vi "pressure_calibration.vi"(10 "calibration":T1(ring), 11 "cmd pressure (mBar)":dbl format="%#_13g") -> (3 "pressure out (mbar)":dbl format="%#_13g")   [LabVIEW 2019]
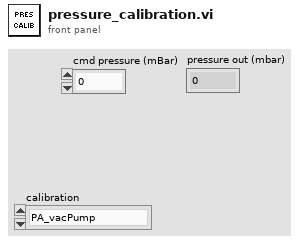
[diagram p1: front panel]
types:
  T1 = enum16{"PA_vacPump", "PA_venturi", "Neuromatics", "ilyaRig", "mightenRig"}
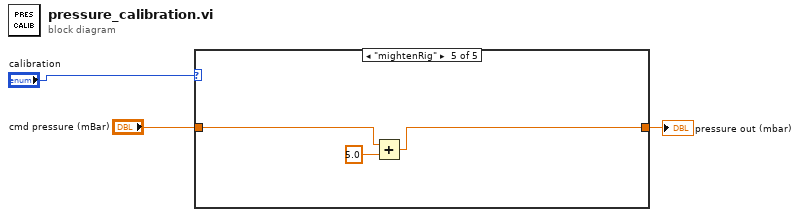
[diagram p0: block diagram]
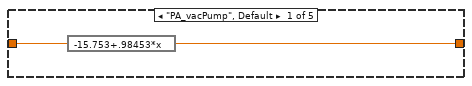
[diagram p2: hidden frame]
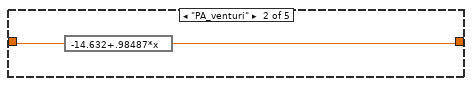
[diagram p3: hidden frame]
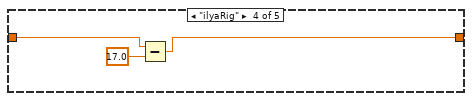
[diagram p5: hidden frame]
diagram:
  n1 = case shown="\"mightenRig\"" "calibration" {
    tunnel: "cmd pressure (mBar)" -> [w5 w7 w8 w11 w13]
    tunnel: [w4 w6 w8 w9 w12] -> w2
    frame "PA_vacPump", Default {
      n2 = expression code="-15.753+.98453*x"(w5) -> (w4:dbl)
    }
    frame "PA_venturi" {
      n3 = expression code="-14.632+.98487*x"(w7) -> (w6:dbl)
    }
    frame "Neuromatics" {
      # "calibration done later on"
    }
    frame "ilyaRig" {
      n4 = Subtract(x=w11, y=17.0) -> (x-y=w9:dbl)
    }
    frame "mightenRig" {
      n5 = Add(x=w13, y=5.0) -> (x+y=w12:dbl)
    }
  }
  "pressure out (mbar)" <- w2
